vi "Write Element of Array Thrusters.vi"(8 "error in (no error)":errorcluster, 9 "Thruster.lvclass":refnum<class "Thruster.lvclass">, 10 "index":i32, 11 "Thrust Allocation in":refnum<class "Thrust Allocation.lvclass">) -> (0 "error out":errorcluster, 3 "Thrust Allocation out":refnum<class "Thrust Allocation.lvclass">)   [LabVIEW 2014, in "Thrust Allocation.lvclass"]
uses:
  Thrust Allocation.lvclass
  Thruster/Thruster.lvclass
  Thrust Allocation.lvclass/Thrust Allocation.ctl
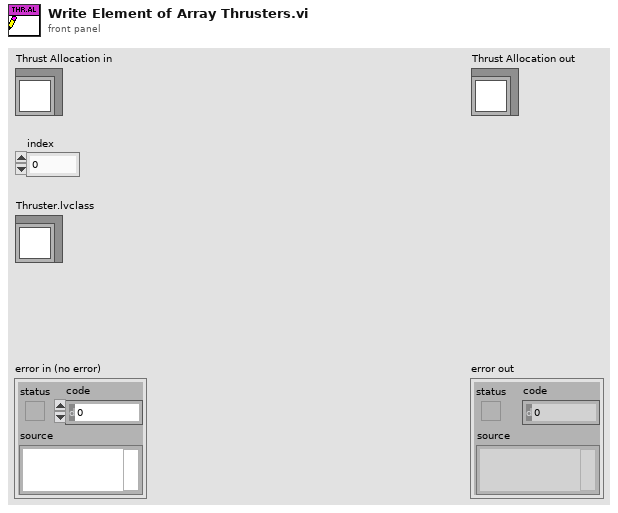
[diagram p1: front panel]
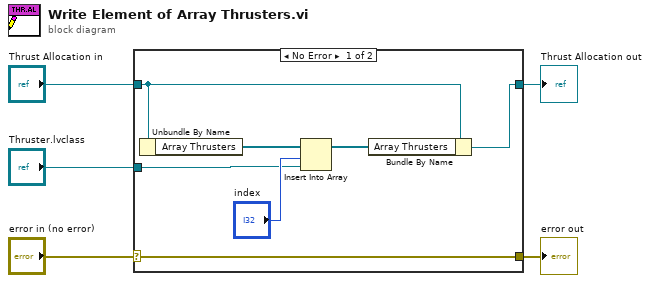
[diagram p0: block diagram]
diagram:
  n1 = case shown="No Error" "error in (no error)" {
    selector: "error in (no error)" -> [w12 w13]
    tunnel: [w12 w13] -> w4
    tunnel: [w11 w14] -> w2
    tunnel: "Thrust Allocation in" -> [w10 w14]
    tunnel: "Thruster.lvclass" -> [w6 _]
    frame No Error {
      n2 = Unbundle By Name(w10) -> ("Array Thrusters"=w9:refnum<class "Thruster.lvclass">[])
      n3 = Insert Into Array(array=w9, index="index", new element=w6) -> (w8:refnum<class "Thruster.lvclass">[])
      n4 = Bundle By Name(cluster=w10, "Array Thrusters"=w8) -> (w11:refnum<class "Thrust Allocation.lvclass">)
    }
    frame Error {
    }
  }
  "error out" <- w4
  "Thrust Allocation out" <- w2
